vi "Mode.vi"(6 "Master Channel (0)":i32, 7 "Set? (F:Read)":bool, 8 "Error In":errorcluster, 9 "Mode (independent)":u16(ring) items=["independent"=0, "slave"=1, "extern"=2, "PCS"=3, "PID"=4, "test"=9], 10 "Channel (0)":i32, 11 "VISA resource name":refnum<visa-resource-name>) -> (0 "Error Out":errorcluster, 3 "dup VISA resource name":refnum<visa-resource-name>, 4 "Master Channel out":i32)   [LabVIEW 2011, in "MGC647C.lvlib"]
doc: "Read/Set mode."
uses:
  <instrlib>/MGC647C/MGC647C.lvlib
panel:
  out "Mode out":u16(ring) items=["independent"=0, "slave"=1, "extern"=2, "PCS"=3, "PID"=4, "test"=9]
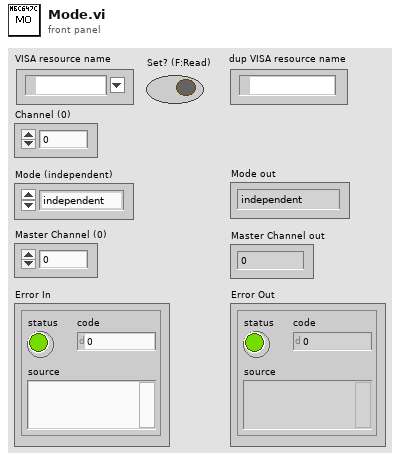
[diagram p1: front panel]
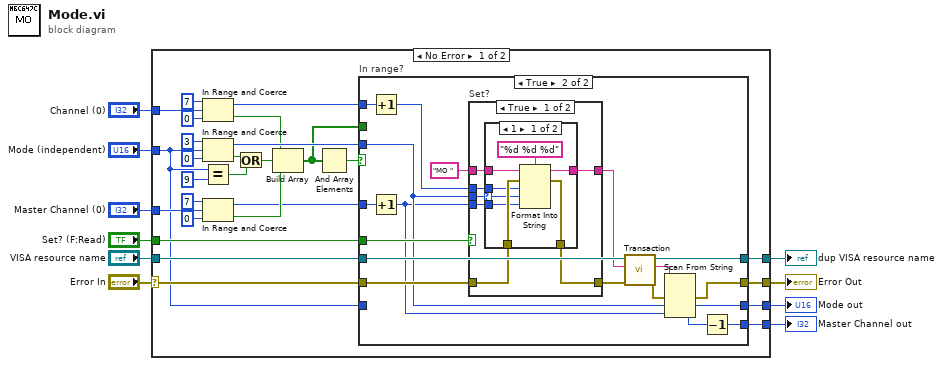
[diagram p0: block diagram]
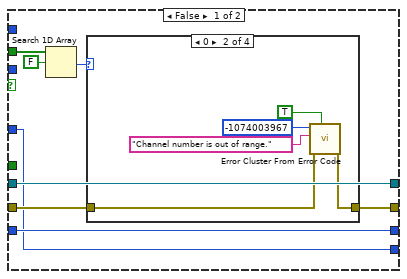
[diagram p2: hidden frame]
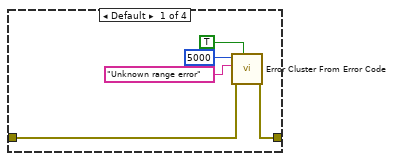
[diagram p3: hidden frame]
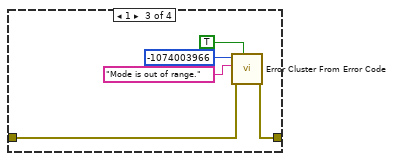
[diagram p4: hidden frame]
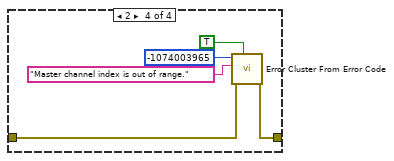
[diagram p5: hidden frame]
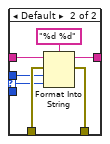
[diagram p6: hidden frame]
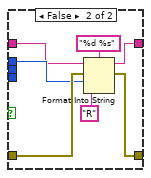
[diagram p7: hidden frame]
diagram:
  n1 = case shown="No Error" "Error In" {
    selector: "Error In" -> [w32 w115]
    tunnel: "VISA resource name" -> [w37 w114]
    tunnel: [w36 w114] -> w9
    tunnel: [w35 w115] -> w8
    tunnel: "Set? (F:Read)" -> [w34 _]
    tunnel: "Mode (independent)" -> [w14 w116]
    tunnel: [w31 w116] -> w1
    tunnel: "Channel (0)" -> [w28 _]
    tunnel: "Master Channel (0)" -> [w17 w113]
    tunnel: [w11 w113] -> w2
    frame No Error {
      n2 = In Range and Coerce(upper limit=7, x=w28, lower limit=0) -> (coerced(x)=w27:i32, In Range?=w26:bool)
      n3 = In Range and Coerce(upper limit=u16 3, x=w14, lower limit=u16 0) -> (coerced(x)=w33:u16, In Range?=w23:bool)
      n4 = Equal?(x=w14, y=u16 9) -> (x = y?=w20:bool)
      n5 = In Range and Coerce(upper limit=7, x=w17, lower limit=0) -> (coerced(x)=w15:i32, In Range?=w16:bool)
      n6 = Or(x=w23, y=w20) -> (x .or. y?=w22:bool)
      n7 = Build Array(w26, w22, w16) -> (w12:bool[])
      n8 = And Array Elements(Boolean array=w12) -> (logical AND=w13:bool)
      n9 = case "In range?" shown="True" w13 {
        tunnel: w37 -> [w43 w83]
        tunnel: [w43 w82] -> w36
        tunnel: [w44 w77] -> w35
        tunnel: w34 -> [_ w72]
        tunnel: w33 -> [_ w69]
        tunnel: w32 -> [w45 w81]
        tunnel: [w42 w71] -> w31
        tunnel: w27 -> [_ w76]
        tunnel: w15 -> [w38 w70]
        tunnel: w14 -> [w42 _]
        tunnel: w12 -> [w41 _]
        tunnel: [w38 w67] -> w11
        frame False {
          n10 = Search 1D Array(1D array=w41, element=FALSE) -> (index of element=w39:i32)  [unwired: 1 in]
          n11 = case shown="0" w39 {
            tunnel: w45 -> [w50 w55 w60 w65]
            tunnel: [w49 w54 w59 w64] -> w44
            frame Default {
              n12 = call <vilib>:"Error Cluster From Error Code.vi"("show call chain? (False)"=TRUE, "error in (no error)"=w50, "error message (\"\")"="Unknown range error" ("error message (\"\")"), "error code (0)"=5000) -> ("error out"=w49:errorcluster)  [unwired: 5 in]
            }
            frame 0 {
              n13 = call <vilib>:"Error Cluster From Error Code.vi"("show call chain? (False)"=TRUE, "error in (no error)"=w55, "error message (\"\")"="Channel number is out of range." ("error message (\"\")"), "error code (0)"=-1074003967) -> ("error out"=w54:errorcluster)  [unwired: 5 in]
            }
            frame 1 {
              n14 = call <vilib>:"Error Cluster From Error Code.vi"("show call chain? (False)"=TRUE, "error in (no error)"=w60, "error message (\"\")"="Mode is out of range." ("error message (\"\")"), "error code (0)"=-1074003966) -> ("error out"=w59:errorcluster)  [unwired: 5 in]
            }
            frame 2 {
              n15 = call <vilib>:"Error Cluster From Error Code.vi"("show call chain? (False)"=TRUE, "error in (no error)"=w65, "error message (\"\")"="Master channel index is out of range." ("error message (\"\")"), "error code (0)"=-1074003965) -> ("error out"=w64:errorcluster)  [unwired: 5 in]
            }
          }
        }
        frame True {
          n16 = Increment(x=w76) -> (x+1=w75:i32)
          n17 = Increment(x=w70) -> (x+1=w66:i32)
          n18 = case "Set?" shown="True" w72 {
            tunnel: w81 -> [w90 w112]
            tunnel: [w89 w111] -> w80
            tunnel: w75 -> [w88 w110]
            tunnel: w69 -> [w85 _]
            tunnel: "MO " ("string (\"\")") -> [w87 w109]
            tunnel: [w86 w108] -> w73
            tunnel: w66 -> [w84 _]
            frame True {
              n19 = case shown="1" w85 {
                selector: w85 -> [w92 w99]
                tunnel: w90 -> [w98 w105]
                tunnel: [w97 w104] -> w89
                tunnel: w88 -> [w96 w103]
                tunnel: w87 -> [w95 w102]
                tunnel: [w94 w101] -> w86
                tunnel: w84 -> [w91 _]
                frame 1 {
                  n20 = Format Into String(format string="%d %d %d", initial string=w95, error in=w98, w96, w92, w91) -> (resulting string=w94:string, error out=w97:errorcluster)
                }
                frame Default {
                  n21 = Format Into String(format string="%d %d", initial string=w102, error in=w105, w103, w99) -> (resulting string=w101:string, error out=w104:errorcluster)
                }
              }
            }
            frame False {
              n22 = Format Into String(format string="%d %s", initial string=w109, error in=w112, w110, "R") -> (resulting string=w108:string, error out=w111:errorcluster)
            }
          }
          n23 = call <instrlib>:"Transaction.vi"("Error In"=w80, "Command"=w73, "VISA resource name"=w83) -> ("Error Out"=w78:errorcluster, "Response"=w79:string, "dup VISA resource name"=w82:refnum<visa-resource-name>)  [unwired: 6 in]
          n24 = Scan From String(input string=w79, error in=w78, default 1=w69, default 2=w66) -> (error out=w77:errorcluster, output 1=w71:u16, output 2=w68:i32)  [unwired: 2 in, 2 out]
          n25 = Decrement(x=w68) -> (x-1=w67:i32)
        }
      }
    }
    frame Error {
    }
  }
  "dup VISA resource name" <- w9
  "Error Out" <- w8
  "Master Channel out" <- w2
  "Mode out" <- w1
